vi "Stop Core.vi"(10 "final error code":i32, 11 "UnitTestEngine In":refnum<class "UnitTestEngine.lvclass">) -> (3 "UnitTestEngine Out":refnum<class "UnitTestEngine.lvclass">)   [LabVIEW 2019, in "UnitTestEngine.lvlib" / "UnitTestEngine.lvclass"]
uses:
  UnitTestEngine.lvclass
  UnitTestEngine.lvclass/UnitTestEngine.ctl
  TestEngine/TestEngine/TestEngine.lvclass
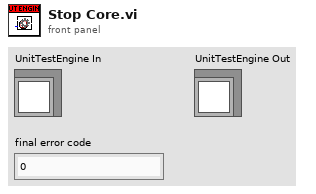
[diagram p1: front panel]
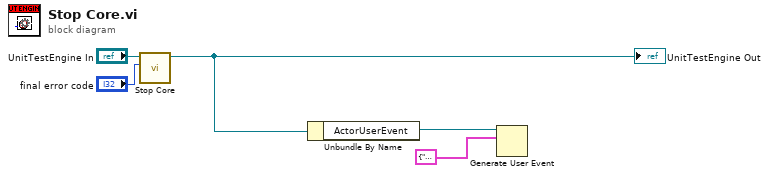
[diagram p0: block diagram]
diagram:
  n1 = call-parent "Stop Core.vi"("final error code"="final error code", "Event Source In"="UnitTestEngine In") -> ("Event Source Out"=w2:refnum<class "UnitTestEngine.lvclass">)  [unwired: 9 in]
  "UnitTestEngine Out" <- w2
  n2 = Unbundle By Name(w2) -> ("ActorUserEvent"=w1:refnum<user-event>)
  n3 = Generate User Event(user event=w1, event data cluster=cluster{"Massage":string, "Value":string} {"Massage"="Exit", "Value"=""} ("event data")) -> ()  [unwired: 2 in, 2 out]
